vi "Get Sub-Item PLC Type.vi"(9 "error in (no error)":errorcluster, 10 ".NET AdsSubItem":refnum<k24>) -> (1 "error out":errorcluster, 2 ".NET AdsSubItem":refnum<k24>, 3 "PLC Type":T1)   [LabVIEW 2018, in "TwinCAT ADS.lvclass"]
uses:
  TwinCAT ADS.lvclass
  TwinCAT.Ads
  Controls/PLC Type.ctl
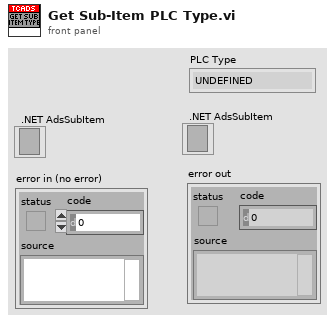
[diagram p1: front panel]
types:
  T1 = typedef "TwinCAT ADS.lvclass/PLC Type.ctl" = enum16{"UNDEFINED", "INT", "DINT", "REAL", "LREAL", "SINT", "BYTE", "UINT", "UDINT", "LINT", "ULINT", "STRING", "WSTRING", "BOOL", "TIME", "LTIME", "DATE", "DT", "TOD", "ARRAY", "JAGGED ARRAY", "STRUCT", "FUNCTION BLOCK", "POINTER", "USER DEFINED"}
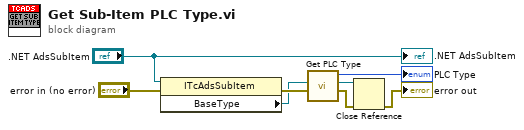
[diagram p0: block diagram]
diagram:
  n1 = property class="ITcAdsSubItem"(reference=".NET AdsSubItem", error in="error in (no error)") -> (error out=w7:errorcluster, "BaseType"=w4:refnum<k24>)  [unwired: 1 out]
  n2 = call "Get PLC Type.vi"("error in (no error)"=w7, ".NET AdsDataType in"=w4) -> ("error out"=w6:errorcluster, ".NET AdsDataType"=w3:refnum<k24>, "PLC Type"=→"PLC Type":T1)  [unwired: 7 in]
  n3 = Close Reference(reference=w3, error in (no error)=w6) -> (error out=→"error out":errorcluster)
  ".NET AdsSubItem" <- ".NET AdsSubItem"
